vi "Netw loop.vi"(8 "error in (no error)":errorcluster, 11 "Queue in":refnum<queue>) -> (0 "error out":errorcluster)   [LabVIEW 2014]
uses:
  Message Queue/Message Cluster.ctl
  Message Queue/Message Queue.lvlib
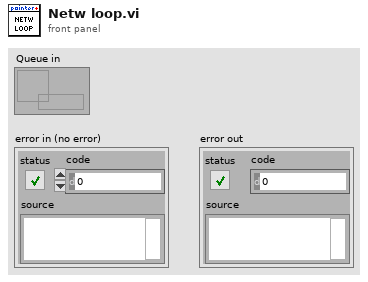
[diagram p1: front panel]
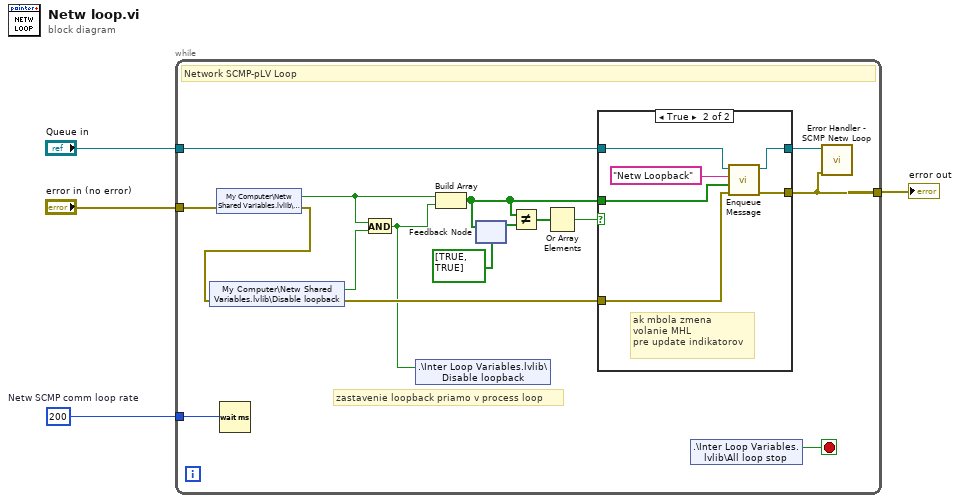
[diagram p0: block diagram]
diagram:
  w1 = u32 200  # Netw SCMP comm loop rate
  n1 = while {
    tunnel: w1 -> [w19]
    tunnel: "Queue in" -> [w15]
    tunnel: "error in (no error)" -> [w18]
    tunnel: [w5] -> w4
    stop <- w20 stop-if-true
    # "zastavenie loopback priamo v process loop"
    # "Network SCMP-pLV Loop"
    n2 = shared-variable "My Computer\\Netw Shared Variables.lvlib\\COMPs"(error in=w18) -> (w12:bool, error out=w17:errorcluster)
    n3 = shared-variable "My Computer\\Netw Shared Variables.lvlib\\Disable loopback"(error in=w17) -> (w16:bool, error out=w13:errorcluster)
    n4 = Wait (ms)(milliseconds to wait=w19) -> ()  [unwired: 1 out]
    n5 = And(x=w12, y=w16) -> (x .and. y?=w11:bool)
    n6 = shared-variable ".\\Inter Loop Variables.lvlib\\Disable loopback"(w11) -> ()  [unwired: 1 in, 1 out]
    n7 = Build Array(w12, w11) -> (w9:bool[])
    n8 = feedback #1(bool[] [TRUE, TRUE]) -> (w10:bool[])
    n9 = feedback-in #1(w9) -> ()
    n10 = Not Equal?(x=w9, y=w10) -> (x != y?=w8:bool[])
    n11 = Or Array Elements(Boolean array=w8) -> (logical OR=w7:bool)
    n12 = case shown="True" w7 {
      tunnel: w15 -> [w22 w27]
      tunnel: [w22 w26] -> w14
      tunnel: w13 -> [w21 w25]
      tunnel: [w21 w24] -> w5
      tunnel: w9 -> [_ w23]
      frame False {
      }
      frame True {
        # "ak mbola zmena\nvolanie MHL\npre update indikatorov"
        n13 = call "Enqueue Message.vi"("error in (no error)"=w25, "Message Data"=w23, "Message"="Netw Loopback", "Message Queue"=w27) -> ("error out"=w24:errorcluster, "dup Message Queue"=w26:refnum<queue>)  [unwired: 6 in]
      }
    }
    n14 = shared-variable ".\\Inter Loop Variables.lvlib\\All loop stop"() -> (w20:bool)  [unwired: 1 in, 1 out]
    n15 = call "Error Handler - SCMP Netw Loop.vi"("error in (no error)"=w5, "Message Queue"=w14) -> ()  [unwired: 9 in, 1 out]
  }
  "error out" <- w4
